vi "Pndt insert carriage return.vi"(1 "transmit script":string="DOF 4\nAMP 1 3\nGAT 1 0 10000\nGAN 1 24\nPRF 200\nSTP 1") -> (4 "display string":string="\r\n", 5 "cmd script":string="\r\n")   [LabVIEW 2026, in "MicroPulse_Driver.lvlib"]
doc: "Replaces line feeds (\\n) from the LabVIEW text box with a carriage return (\\r) termination required by MicroPulse, and removes # tagged lines and AG commands from script files."
uses:
  MicroPulse_Driver.lvlib
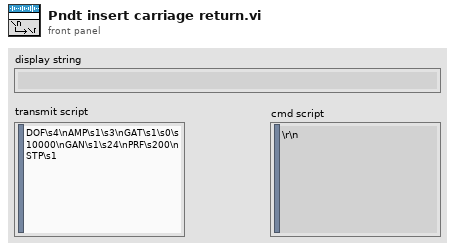
[diagram p1: front panel]
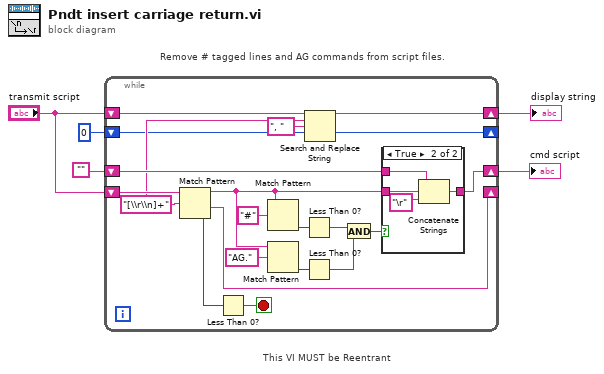
[diagram p0: block diagram]
diagram:
  # "This VI MUST be Reentrant"
  # "Remove # tagged lines and AG commands from script files."
  n1 = while {
    shift-right: [w22] -> w2
    shift-left: "" -> [w21]
    shift-right: [w23] -> _
    shift-left: "transmit script" -> [w24]
    shift-right: [w18] -> w1
    shift-left: "transmit script" -> [w20]
    shift-right: [w16] -> _
    shift-left: 0 ("offset past replacement") -> [w17]
    stop <- w15 stop-if-true
    w19 = "[\\r\\n]+" ("regular expression")
    n2 = Match Pattern(string=w24, regular expression=w19) -> (before substring=w8:string, after substring=w23:string, offset past match=w25:i32)  [unwired: 1 in, 1 out]
    n3 = Less Than 0?(x=w25) -> (x < 0?=w15:bool)
    n4 = Match Pattern(string=w8, regular expression="#") -> (offset past match=w12:i32)  [unwired: 1 in, 3 out]
    n5 = Match Pattern(string=w8, regular expression="AG.") -> (offset past match=w10:i32)  [unwired: 1 in, 3 out]
    n6 = Less Than 0?(x=w12) -> (x < 0?=w6:bool)
    n7 = Less Than 0?(x=w10) -> (x < 0?=w7:bool)
    n8 = Search and Replace String(input string=w20, search string=w19, replace string=", " ("replace string (\"\")"), offset=w17) -> (result string=w18:string, offset past replacement=w16:i32)  [unwired: 4 in, 2 out]
    n9 = And(x=w6, y=w7) -> (x .and. y?=w11:bool)
    n10 = case shown="True" w11 {
      tunnel: [w26 w29] -> w22
      tunnel: w21 -> [w26 w28]
      tunnel: w8 -> [_ w27]
      frame False {
      }
      frame True {
        n11 = Concatenate Strings(w28, w27, "\r" ("regular expression")) -> (w29:string)
      }
    }
  }
  "cmd script" <- w2
  "display string" <- w1
